vi "Measurement UI.vi"() -> ()   [LabVIEW 2025, in "TDMS Waveform Creator UI.lvlib"]
uses:
  TDMS Waveform Creator UI.lvlib
panel:
  out "Wfm List Item When Drag Start":i32
  out "Waveform Preview (Canvas)":waveform(dbl)(graph)
  in  "Waveform List":i32(listbox)
  in  "Duration":dbl=0.002 format="%#_6ps"
  in  "Sample Rate":dbl=10000000.0 caption="Sample Rate (Resampled)" format="%#_6pHz"
  in  "Add to Save":bool
  in  "Clear All":bool
  in  "Waveforms Summary JSON":string[](array[string])
  out "Waveform Preview (To Save)":waveform(dbl)[](graph)
  out "Channels Item When Drag Start":i32
  out "Max Sample Rate":dbl format="%#_6pHz"
  in  "Channel Names":string[](array[string])
  in  "Run Action":string(combo)="Create/Replace Wfm Group"
  in  "TDMS File Location":path
  in  "Wfm Group Name":string="Wfm1"
  in  "Channels":i32(listbox)
  # "Canvas"
  # "Waveform Group to Save"
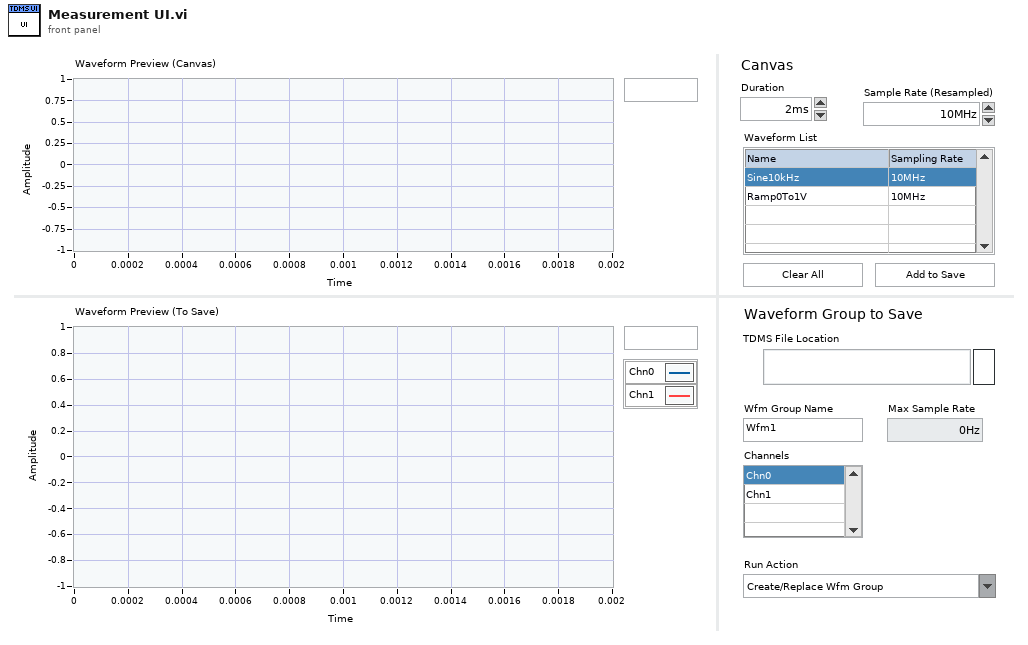
[diagram p1: front panel]
types:
  T1 = cluster{"Canvas Wfm Array":waveform(dbl)[], "To Save Wfm Arrays":waveform(dbl)[]}
  T2 = cluster{"Channels":refnum<vi>, "Channel Names":refnum<vi>, "Waveform Preview (To Save)":refnum<vi>, "Waveforms Summary JSON":refnum<vi>, "Max Sample Rate":refnum<vi>}
  T3 = cluster{"Waveform List":refnum<vi>, "Duration":refnum<vi>, "Sample Rate":refnum<vi>}
  T4 = enum16{"No Item", "1 Item", ">2 Item", "Invalid Selection"}
  T5 = typedef "LVPoint32TypeDef.ctl" = cluster{"Horizontal":i32, "Vertical":i32}
  T6 = typedef "LVRowAndColumnTypeDef.ctl" = cluster{"Row":i32, "Column":i32}
  T7 = cluster{"Canvas Wfm Array Out":waveform(dbl)[], "To Save Wfm Arrays":waveform(dbl)[]}
  T8 = cluster{"Channel Names":string[], "To Save Wfm Arrays Out":waveform(dbl)[], "Waveform Summary JSON":string[]}
  T9 = cluster{"Channel Names":string[], "To Save Wfm Arrays":waveform(dbl)[], "Waveform Summary JSON":string[]}
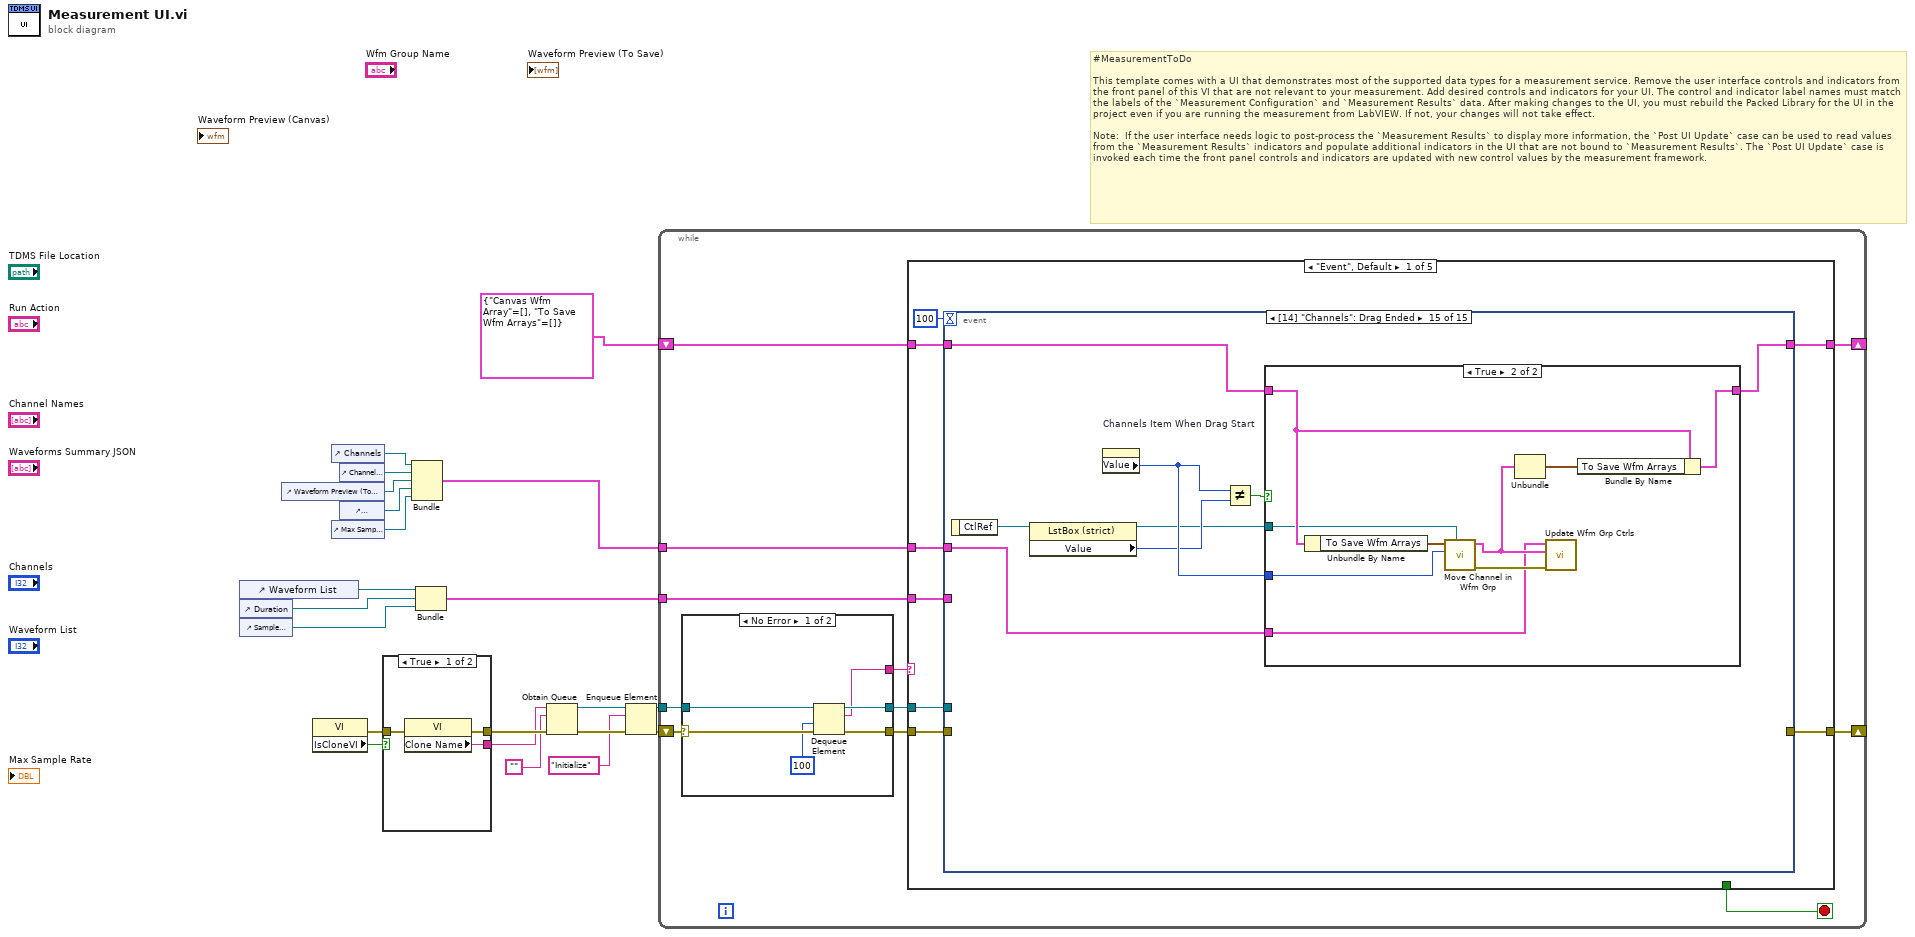
[diagram p0: block diagram]
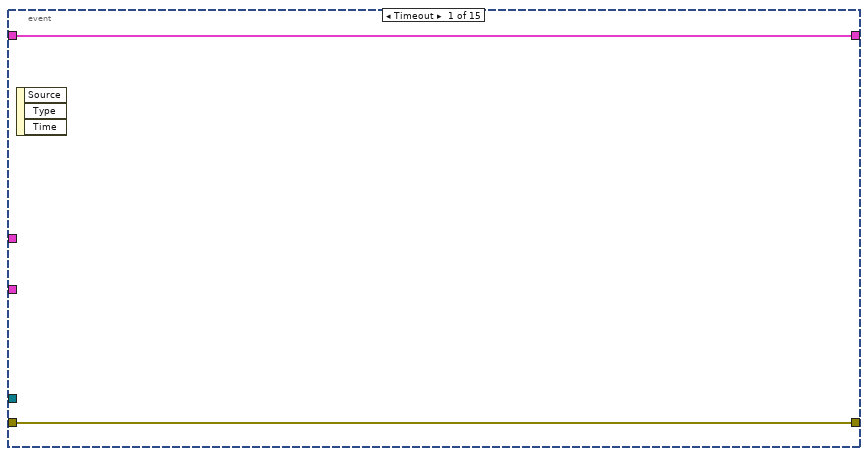
[diagram p2: hidden frame]
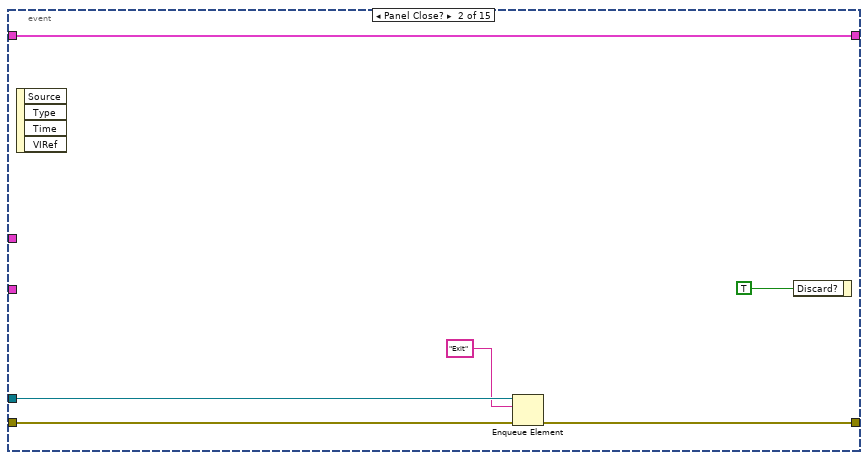
[diagram p3: hidden frame]
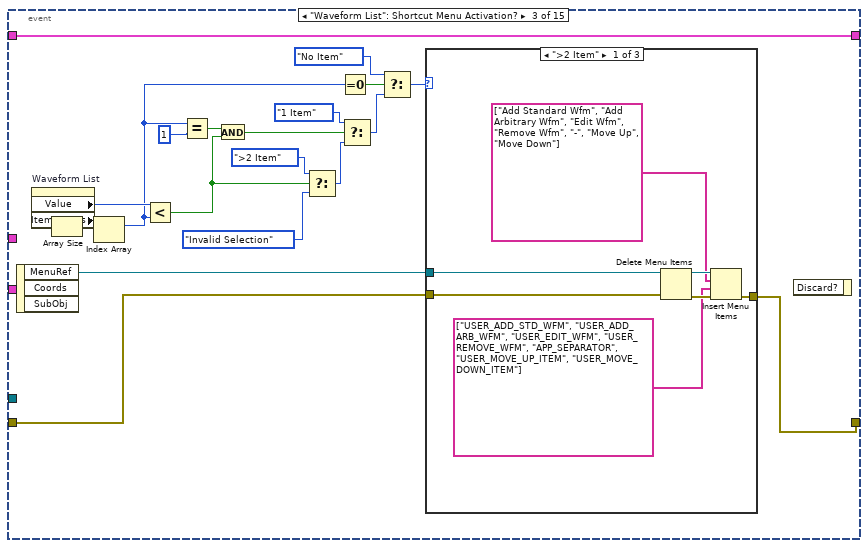
[diagram p4: hidden frame]
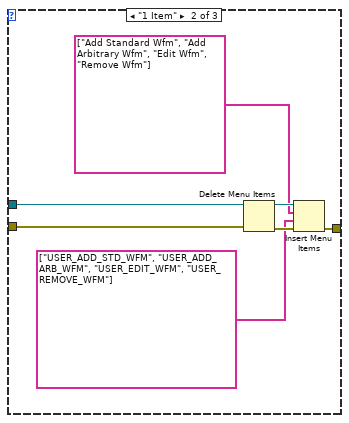
[diagram p5: hidden frame]
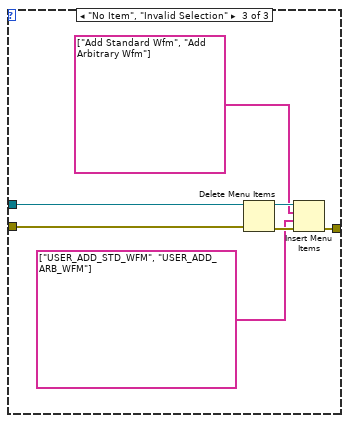
[diagram p6: hidden frame]
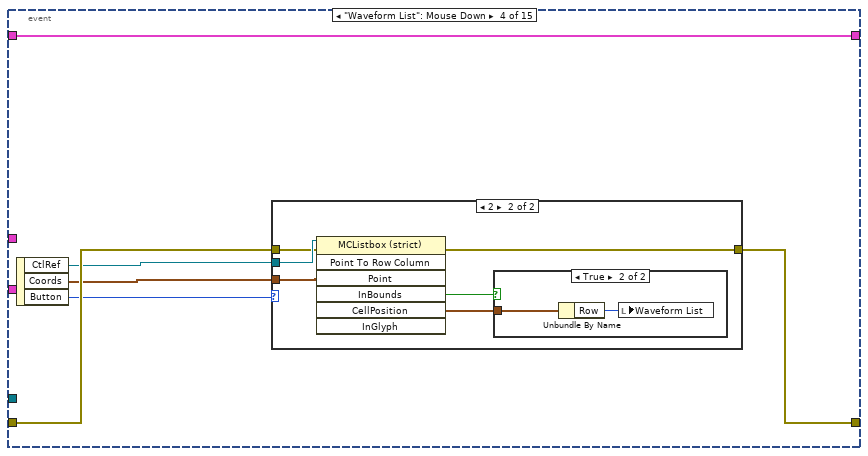
[diagram p7: hidden frame]
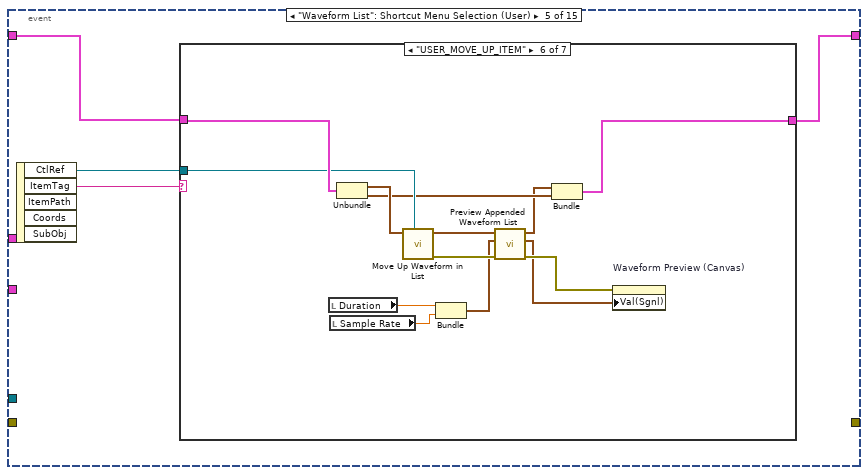
[diagram p10: hidden frame]
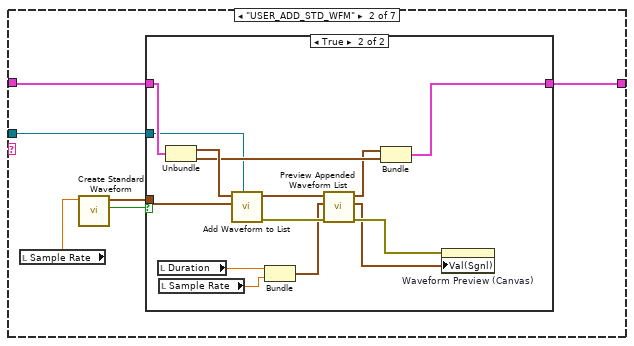
[diagram p12: hidden frame]
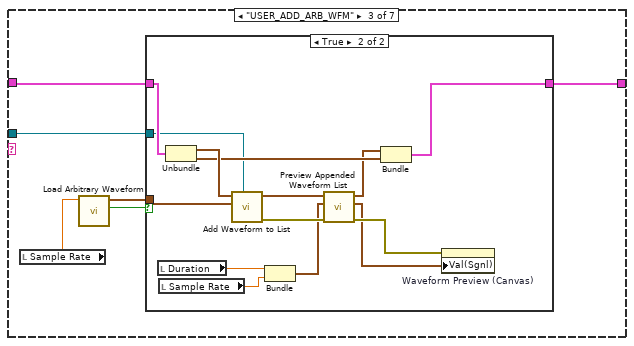
[diagram p14: hidden frame]
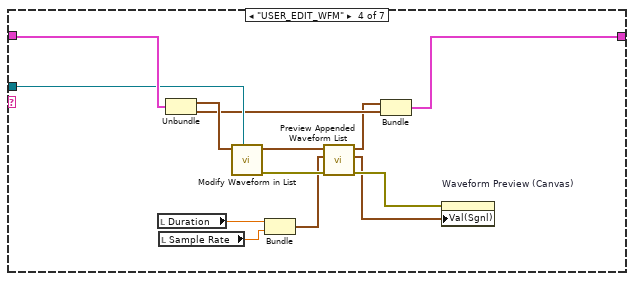
[diagram p16: hidden frame]
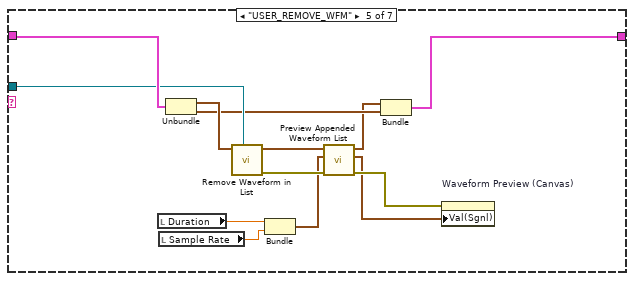
[diagram p17: hidden frame]
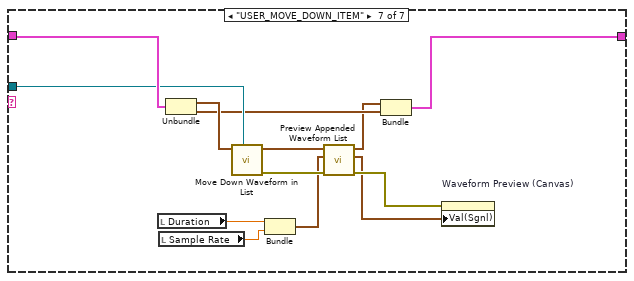
[diagram p18: hidden frame]
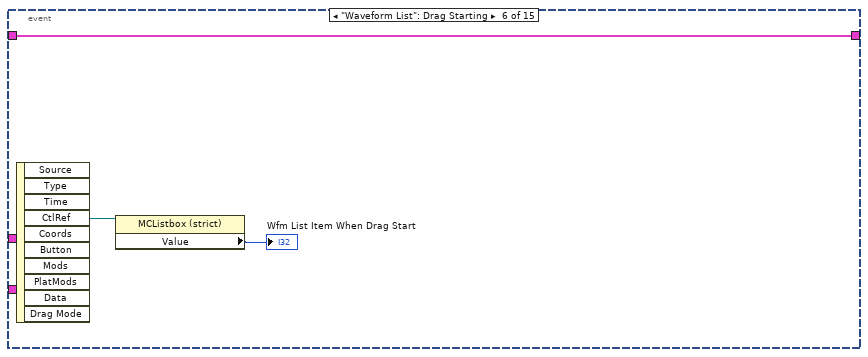
[diagram p19: hidden frame]
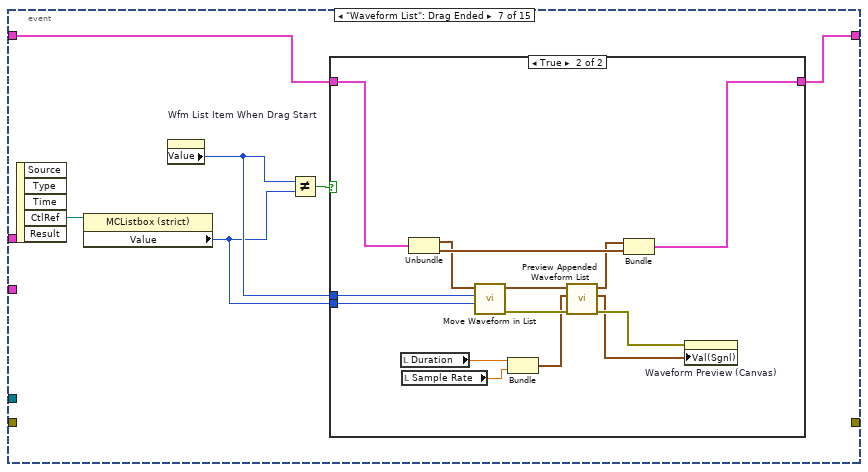
[diagram p20: hidden frame]
diagram:
  # "#MeasurementToDo  \n\nThis template comes with a UI that demonstrates most of the supported data types for a measurement service. Remove the user interface controls and indicators from the front panel of this VI that are not relevant to your measurement. Add desired controls and indicators for your UI. The control and indicator label names must match the labels of the `Measurement Configuration` and `Measurement Results` data. After making changes to the UI, you must rebuild the Packed Library for the UI in the project even if you are running the measurement from LabVIEW. If not, your changes will not take effect.\n\nNote:  If the user interface needs logic to post-process the `Measurement Results` to display more information, the `Post UI Update` case can be used to read values from the `Measurement Results` indicators and populate additional indicators in the UI that are not bound to `Measurement Results`. The `Post UI Update` case is invoked each time the front panel controls and indicators are updated with new control values by the measurement framework."
  n1 = control-ref of="Waveform List"() -> (w4:refnum<vi>)
  n2 = control-ref of="Duration"() -> (w5:refnum<vi>)
  n3 = control-ref of="Sample Rate"() -> (w6:refnum<vi>)
  n4 = control-ref of="Waveform Preview (To Save)"() -> (w8:refnum<vi>)
  n5 = property class="VI"() -> (error out=w12:errorcluster, "IsCloneVI"=w13:bool)  [unwired: 2 in, 1 out]
  n6 = control-ref of="Channels"() -> (w1:refnum<vi>)
  n7 = control-ref of="Max Sample Rate"() -> (w10:refnum<vi>)
  n8 = control-ref of="Channel Names"() -> (w7:refnum<vi>)
  n9 = control-ref of="Waveforms Summary JSON"() -> (w9:refnum<vi>)
  n10 = case shown="True" w13 {
    tunnel: [w24 w27] -> w21
    tunnel: [w23 w26] -> w20
    tunnel: w12 -> [w22 w25]
    frame True {
      n11 = property class="VI"(error in=w22) -> (error out=w24:errorcluster, "Clone Name"=w23:string)  [unwired: 1 in, 1 out]
    }
    frame False {
      n12 = property class="VI"(error in=w25) -> (error out=w27:errorcluster, "Name"=w26:string)  [unwired: 1 in, 1 out]
    }
  }
  n13 = Bundle("Channels"=w1, "Channel Names"=w7, "Waveform Preview (To Save)"=w8, "Waveforms Summary JSON"=w9, "Max Sample Rate"=w10) -> (w3:T2)  [unwired: 1 in]
  n14 = Bundle("Waveform List"=w4, "Duration"=w5, "Sample Rate"=w6) -> (w2:T3)  [unwired: 1 in]
  n15 = Obtain Queue(name (unnamed)=w20, element data type="", error in (no error)=w21) -> (queue out=w17:refnum<queue>, error out=w19:errorcluster)  [unwired: 2 in, 1 out]
  n16 = Enqueue Element(queue=w17, element="Initialize", error in (no error)=w19) -> (queue out=w16:refnum<queue>, error out=w18:errorcluster)  [unwired: 1 in, 1 out]
  n17 = while {
    shift-right: [w33] -> _
    shift-left: w18 -> [w38]
    tunnel: w16 -> [w36]
    shift-right: [w31] -> _
    shift-left: T1 {"Canvas Wfm Array"=[], "To Save Wfm Arrays"=[]} -> [w30]
    tunnel: w3 -> [w29]
    tunnel: w2 -> [w28]
    stop <- w32 stop-if-true
    n18 = case shown="No Error" w38 {
      selector: w38 -> [w459 w462]
      tunnel: [w458 w462] -> w37
      tunnel: w36 -> [w457 w461]
      tunnel: [w456 w461] -> w35
      tunnel: [w455 "Handle Error"] -> w34
      frame No Error {
        n19 = Dequeue Element(queue=w457, timeout in ms (-1)=100, error in (no error)=w459) -> (queue out=w456:refnum<queue>, element=w455:string, error out=w458:errorcluster)  [unwired: 1 out]
      }
      frame Error {
      }
    }
    n20 = case shown="\"Event\", Default" w34 {
      tunnel: w37 -> [w45 w433 w438 w451 w453]
      tunnel: w35 -> [w43 _ _ w449 _]
      tunnel: [w46 w429 w442 w446 w453] -> w33
      tunnel: [_ FALSE _ TRUE _] -> w32
      tunnel: [w42 w430 w440 w444 w452] -> w31
      tunnel: w30 -> [w41 w430 w443 w444 w452]
      tunnel: w29 -> [w40 _ w441 _ _]
      tunnel: w28 -> [w39 _ _ _ _]
      frame "Event", Default {
        n21 = event shown="[14] \"Channels\": Drag Ended" {
          selector: _ -> [_ _ _ _ _ _ _ _ _ _ _ _ _ _ _]
          dyn-events: _ -> [_ _ _ _ _ _ _ _ _ _ _ _ _ _ _]
          timeout: 100 -> [_ _ _ _ _ _ _ _ _ _ _ _ _ _ _]
          tunnel: [w48 w52 w73 w97 _ _ _ w236 w246 w259 w299 w324 w341 _ _] -> w46
          tunnel: w45 -> [w48 w53 w74 w101 _ _ _ w235 w245 w263 w300 w328 w339 _ _]
          tunnel: w43 -> [_ w51 _ _ _ _ _ _ _ _ _ _ _ _ _]
          tunnel: [w47 w49 w72 w96 w112 w212 w215 w239 w254 w264 w298 w323 w342 w410 w415] -> w42
          tunnel: w41 -> [w47 w49 w72 w96 w111 w212 w216 w239 w255 w262 w298 w323 w340 w410 w416]
          tunnel: w40 -> [_ _ _ _ _ _ _ _ _ w256 _ _ w338 _ w412]
          tunnel: w39 -> [_ _ _ _ _ _ _ _ _ _ _ _ w337 _ _]
          event Timeout {
            n22 = event-data() -> ()  [unwired: 1 in, 3 out]
          }
          event Panel Close? {
            n23 = event-data() -> ()  [unwired: 1 in, 4 out]
            n24 = Enqueue Element(queue=w51, element="Exit", error in (no error)=w53) -> (error out=w52:errorcluster)  [unwired: 1 in, 2 out]
            n25 = event-data("Discard?"=TRUE) -> ()  [unwired: 1 in, 1 out]
          }
          event "Waveform List": Shortcut Menu Activation? {
            n26 = event-data() -> ("MenuRef"=w68:refnum<k9>)  [unwired: 1 in, 2 out]
            n27 = property on="Waveform List" class="MCListbox (strict)"() -> ("Value"=w70:i32, "ItemNames"=w71:string[][])  [unwired: 2 in, 2 out]
            n28 = Array Size(array=w71) -> (size(s)=w69:i32[])
            n29 = Index Array(array=w69) -> (element=w64:i32)  [unwired: 1 in]
            n30 = Less?(x=w70, y=w64) -> (x < y?=w57:bool)
            n31 = Equal?(x=w64, y=1) -> (x = y?=w62:bool)
            n32 = And(x=w62, y=w57) -> (x .and. y?=w61:bool)
            n33 = Select(t=T4.">2 Item", s=w57, f=T4."Invalid Selection") -> (s? t:f=w59:T4)
            n34 = Equal To 0?(x=w64) -> (x = 0?=w67:bool)
            n35 = Select(t=T4."1 Item", s=w61, f=w59) -> (s? t:f=w56:T4)
            n36 = Select(t=T4."No Item", s=w67, f=w56) -> (s? t:f=w55:T4)
            n37 = case shown="\">2 Item\"" w55 {
              tunnel: w74 -> [w77 w84 w91]
              tunnel: [w76 w83 w90] -> w73
              tunnel: w68 -> [w75 w82 w89]
              frame ">2 Item" {
                n38 = Delete Menu Items(6:w77, 9:w75) -> (0:w81:errorcluster, 3:w80:refnum<k9>)  [unwired: 2 in]
                n39 = Insert Menu Items(6:w81, 7:string[] ["USER_ADD_STD_WFM", "USER_ADD_ARB_WFM", "USER_EDIT_WFM", "USER_REMOVE_WFM", "APP_SEPARATOR", "USER_MOVE_UP_ITEM", "USER_MOVE_DOWN_ITEM"], 8:string[] ["Add Standard Wfm", "Add Arbitrary Wfm", "Edit Wfm", "Remove Wfm", "-", "Move Up", "Move Down"], 9:w80) -> (0:w76:errorcluster)  [unwired: 2 in, 2 out]
              }
              frame "1 Item" {
                n40 = Delete Menu Items(6:w84, 9:w82) -> (0:w88:errorcluster, 3:w87:refnum<k9>)  [unwired: 2 in]
                n41 = Insert Menu Items(6:w88, 7:string[] ["USER_ADD_STD_WFM", "USER_ADD_ARB_WFM", "USER_EDIT_WFM", "USER_REMOVE_WFM"], 8:string[] ["Add Standard Wfm", "Add Arbitrary Wfm", "Edit Wfm", "Remove Wfm"], 9:w87) -> (0:w83:errorcluster)  [unwired: 2 in, 2 out]
              }
              frame "No Item", "Invalid Selection" {
                n42 = Delete Menu Items(6:w91, 9:w89) -> (0:w95:errorcluster, 3:w94:refnum<k9>)  [unwired: 2 in]
                n43 = Insert Menu Items(6:w95, 7:string[] ["USER_ADD_STD_WFM", "USER_ADD_ARB_WFM"], 8:string[] ["Add Standard Wfm", "Add Arbitrary Wfm"], 9:w94) -> (0:w90:errorcluster)  [unwired: 2 in, 2 out]
              }
            }
            n44 = event-data() -> ()  [unwired: 2 in, 1 out]
          }
          event "Waveform List": Mouse Down {
            n45 = event-data() -> ("CtlRef"=w100:refnum<vi>, "Coords"=w99:T5, "Button"=w98:u16)  [unwired: 1 in]
            n46 = case shown="2" w98 {
              tunnel: w99 -> [_ w108]
              tunnel: w100 -> [_ w107]
              tunnel: w101 -> [w102 w105]
              tunnel: [w102 w106] -> w97
              frame Default {
              }
              frame 2 {
                n47 = invoke class="MCListbox (strict)" method="Point To Row Column"(reference=w107, error in=w105, "Point"=w108) -> (error out=w106:errorcluster, "InBounds"=w103:bool, "CellPosition"=w104:T6)  [unwired: 4 in, 4 out]
                n48 = case shown="True" w103 {
                  tunnel: w104 -> [_ w110]
                  frame False {
                  }
                  frame True {
                    n49 = Unbundle By Name(w110) -> ("Row"=w109:i32)
                    n50 = local write "Waveform List"(w109) -> ()
                  }
                }
              }
            }
          }
          event "Waveform List": Shortcut Menu Selection (User) {
            n51 = event-data() -> ("CtlRef"=w113:refnum<vi>, "ItemTag"=w114:string)  [unwired: 1 in, 3 out]
            n52 = case shown="\"USER_MOVE_UP_ITEM\"" w114 {
              tunnel: w113 -> [_ w117 w138 w168 w181 w194 w207]
              tunnel: [w115 w121 w142 w170 w183 w196 w209] -> w112
              tunnel: w111 -> [w115 w118 w139 w169 w182 w195 w208]
              frame Default {
              }
              frame "USER_ADD_STD_WFM" {
                n53 = local read "Sample Rate"() -> (w116:dbl)
                n54 = call "Create Standard Waveform.vi"("Suggested Sample Rate (Hz)"=w116) -> ("Waveform Created?"=w120:bool, "Output Waveform"=w119:waveform(dbl))  [unwired: 9 in]
                n55 = case shown="True" w120 {
                  tunnel: [w122 w133] -> w121
                  tunnel: w119 -> [_ w136]
                  tunnel: w118 -> [w122 w135]
                  tunnel: w117 -> [_ w129]
                  frame False {
                  }
                  frame True {
                    n56 = local read "Duration"() -> (w131:dbl)
                    n57 = local read "Sample Rate"() -> (w130:dbl)
                    n58 = Unbundle(w135) -> ("Canvas Wfm Array"=w134:waveform(dbl)[], "To Save Wfm Arrays"=w132:waveform(dbl)[])
                    n59 = call "Add Waveform to List.vi"("Waveform List Ctl Ref"=w129, "Waveform to Add"=w136, "Canvas Wfm Array In"=w134) -> ("error out"=w128:errorcluster, "Canvas Wfm Array Out"=w126:waveform(dbl)[])  [unwired: 7 in]
                    n60 = Bundle("Duration"=w131, "Sample Rate"=w130) -> (w123:cluster{"Duration":dbl, "Sample Rate":dbl})  [unwired: 1 in]
                    n61 = call "Preview Appended Waveform List.vi"("error in (no error)"=w128, "Trim and Resample Settings"=w123, "Canvas Wfm Array In"=w126) -> ("error out"=w127:errorcluster, "Final Waveform"=w124:waveform(dbl), "Canvas Wfm Array Out"=w125:waveform(dbl)[])  [unwired: 6 in]
                    n62 = Bundle("Canvas Wfm Array Out"=w125, "To Save Wfm Arrays"=w132) -> (w133:T7)  [unwired: 1 in]
                    n63 = property on="Waveform Preview (Canvas)" class="WFGraph (strict)"(error in=w127, "Val(Sgnl)"=w124) -> ()  [unwired: 1 in, 2 out]
                  }
                }
              }
              frame "USER_ADD_ARB_WFM" {
                n64 = local read "Sample Rate"() -> (w137:dbl)
                n65 = call "Load Arbitrary Waveform.vi"("Suggested Sample Rate"=w137) -> ("Waveform Created?"=w141:bool, "Output Waveform"=w140:waveform(dbl))  [unwired: 9 in]
                n66 = case shown="True" w141 {
                  tunnel: [w143 w154] -> w142
                  tunnel: w140 -> [_ w157]
                  tunnel: w139 -> [w143 w156]
                  tunnel: w138 -> [_ w150]
                  frame False {
                  }
                  frame True {
                    n67 = local read "Duration"() -> (w152:dbl)
                    n68 = local read "Sample Rate"() -> (w151:dbl)
                    n69 = Unbundle(w156) -> ("Canvas Wfm Array"=w155:waveform(dbl)[], "To Save Wfm Arrays"=w153:waveform(dbl)[])
                    n70 = call "Add Waveform to List.vi"("Waveform List Ctl Ref"=w150, "Waveform to Add"=w157, "Canvas Wfm Array In"=w155) -> ("error out"=w149:errorcluster, "Canvas Wfm Array Out"=w147:waveform(dbl)[])  [unwired: 7 in]
                    n71 = Bundle("Duration"=w152, "Sample Rate"=w151) -> (w144:cluster{"Duration":dbl, "Sample Rate":dbl})  [unwired: 1 in]
                    n72 = call "Preview Appended Waveform List.vi"("error in (no error)"=w149, "Trim and Resample Settings"=w144, "Canvas Wfm Array In"=w147) -> ("error out"=w148:errorcluster, "Final Waveform"=w145:waveform(dbl), "Canvas Wfm Array Out"=w146:waveform(dbl)[])  [unwired: 6 in]
                    n73 = Bundle("Canvas Wfm Array Out"=w146, "To Save Wfm Arrays"=w153) -> (w154:T7)  [unwired: 1 in]
                    n74 = property on="Waveform Preview (Canvas)" class="WFGraph (strict)"(error in=w148, "Val(Sgnl)"=w145) -> ()  [unwired: 1 in, 2 out]
                  }
                }
              }
              frame "USER_EDIT_WFM" {
                n75 = local read "Duration"() -> (w165:dbl)
                n76 = local read "Sample Rate"() -> (w164:dbl)
                n77 = Unbundle(w169) -> ("Canvas Wfm Array"=w167:waveform(dbl)[], "To Save Wfm Arrays"=w166:waveform(dbl)[])
                n78 = call "Modify Waveform in List.vi"("Waveform List Ctl Ref"=w168, "Canvas Wfm Array In"=w167) -> ("error out"=w163:errorcluster, "Canvas Wfm Array Out"=w161:waveform(dbl)[])  [unwired: 8 in]
                n79 = Bundle("Duration"=w165, "Sample Rate"=w164) -> (w158:cluster{"Duration":dbl, "Sample Rate":dbl})  [unwired: 1 in]
                n80 = call "Preview Appended Waveform List.vi"("error in (no error)"=w163, "Trim and Resample Settings"=w158, "Canvas Wfm Array In"=w161) -> ("error out"=w162:errorcluster, "Final Waveform"=w159:waveform(dbl), "Canvas Wfm Array Out"=w160:waveform(dbl)[])  [unwired: 6 in]
                n81 = Bundle("Canvas Wfm Array Out"=w160, "To Save Wfm Arrays"=w166) -> (w170:T7)  [unwired: 1 in]
                n82 = property on="Waveform Preview (Canvas)" class="WFGraph (strict)"(error in=w162, "Val(Sgnl)"=w159) -> ()  [unwired: 1 in, 2 out]
              }
              frame "USER_REMOVE_WFM" {
                n83 = local read "Duration"() -> (w178:dbl)
                n84 = local read "Sample Rate"() -> (w177:dbl)
                n85 = Unbundle(w182) -> ("Canvas Wfm Array"=w180:waveform(dbl)[], "To Save Wfm Arrays"=w179:waveform(dbl)[])
                n86 = call "Remove Waveform in List.vi"("Waveform List Ctl Ref"=w181, "Canvas Wfm Array In"=w180) -> ("error out"=w176:errorcluster, "Canvas Wfm Array Out"=w174:waveform(dbl)[])  [unwired: 8 in]
                n87 = Bundle("Duration"=w178, "Sample Rate"=w177) -> (w171:cluster{"Duration":dbl, "Sample Rate":dbl})  [unwired: 1 in]
                n88 = call "Preview Appended Waveform List.vi"("error in (no error)"=w176, "Trim and Resample Settings"=w171, "Canvas Wfm Array In"=w174) -> ("error out"=w175:errorcluster, "Final Waveform"=w172:waveform(dbl), "Canvas Wfm Array Out"=w173:waveform(dbl)[])  [unwired: 6 in]
                n89 = Bundle("Canvas Wfm Array Out"=w173, "To Save Wfm Arrays"=w179) -> (w183:T7)  [unwired: 1 in]
                n90 = property on="Waveform Preview (Canvas)" class="WFGraph (strict)"(error in=w175, "Val(Sgnl)"=w172) -> ()  [unwired: 1 in, 2 out]
              }
              frame "USER_MOVE_UP_ITEM" {
                n91 = local read "Duration"() -> (w191:dbl)
                n92 = local read "Sample Rate"() -> (w190:dbl)
                n93 = Unbundle(w195) -> ("Canvas Wfm Array"=w193:waveform(dbl)[], "To Save Wfm Arrays"=w192:waveform(dbl)[])
                n94 = call "Move Up Waveform in List.vi"("Waveform List Ctl Ref"=w194, "Canvas Wfm Array In"=w193) -> ("error out"=w189:errorcluster, "Canvas Wfm Array Out"=w187:waveform(dbl)[])  [unwired: 8 in]
                n95 = Bundle("Duration"=w191, "Sample Rate"=w190) -> (w184:cluster{"Duration":dbl, "Sample Rate":dbl})  [unwired: 1 in]
                n96 = call "Preview Appended Waveform List.vi"("error in (no error)"=w189, "Trim and Resample Settings"=w184, "Canvas Wfm Array In"=w187) -> ("error out"=w188:errorcluster, "Final Waveform"=w185:waveform(dbl), "Canvas Wfm Array Out"=w186:waveform(dbl)[])  [unwired: 6 in]
                n97 = Bundle("Canvas Wfm Array Out"=w186, "To Save Wfm Arrays"=w192) -> (w196:T7)  [unwired: 1 in]
                n98 = property on="Waveform Preview (Canvas)" class="WFGraph (strict)"(error in=w188, "Val(Sgnl)"=w185) -> ()  [unwired: 1 in, 2 out]
              }
              frame "USER_MOVE_DOWN_ITEM" {
                n99 = local read "Duration"() -> (w204:dbl)
                n100 = local read "Sample Rate"() -> (w203:dbl)
                n101 = Unbundle(w208) -> ("Canvas Wfm Array"=w206:waveform(dbl)[], "To Save Wfm Arrays"=w205:waveform(dbl)[])
                n102 = call "Move Down Waveform in List.vi"("Waveform List Ctl Ref"=w207, "Canvas Wfm Array In"=w206) -> ("error out"=w202:errorcluster, "Canvas Wfm Array Out"=w200:waveform(dbl)[])  [unwired: 8 in]
                n103 = Bundle("Duration"=w204, "Sample Rate"=w203) -> (w197:cluster{"Duration":dbl, "Sample Rate":dbl})  [unwired: 1 in]
                n104 = call "Preview Appended Waveform List.vi"("error in (no error)"=w202, "Trim and Resample Settings"=w197, "Canvas Wfm Array In"=w200) -> ("error out"=w201:errorcluster, "Final Waveform"=w198:waveform(dbl), "Canvas Wfm Array Out"=w199:waveform(dbl)[])  [unwired: 6 in]
                n105 = Bundle("Canvas Wfm Array Out"=w199, "To Save Wfm Arrays"=w205) -> (w209:T7)  [unwired: 1 in]
                n106 = property on="Waveform Preview (Canvas)" class="WFGraph (strict)"(error in=w201, "Val(Sgnl)"=w198) -> ()  [unwired: 1 in, 2 out]
              }
            }
          }
          event "Waveform List": Drag Starting {
            n107 = event-data() -> ("CtlRef"=w211:refnum<vi>)  [unwired: 1 in, 9 out]
            n108 = property class="MCListbox (strict)"(reference=w211) -> ("Value"=→"Wfm List Item When Drag Start":i32)  [unwired: 1 in, 2 out]
          }
          event "Waveform List": Drag Ended {
            n109 = event-data() -> ("CtlRef"=w218:refnum<vi>)  [unwired: 1 in, 4 out]
            n110 = property class="MCListbox (strict)"(reference=w218) -> ("Value"=w213:i32)  [unwired: 1 in, 2 out]
            n111 = property on="Wfm List Item When Drag Start" class="DigNum (strict)"() -> ("Value"=w214:i32)  [unwired: 2 in, 2 out]
            n112 = Not Equal?(x=w214, y=w213) -> (x != y?=w217:bool)
            n113 = case shown="True" w217 {
              tunnel: w216 -> [w219 w224]
              tunnel: [w219 w223] -> w215
              tunnel: w214 -> [_ w221]
              tunnel: w213 -> [_ w220]
              frame False {
              }
              frame True {
                n114 = local read "Duration"() -> (w232:dbl)
                n115 = local read "Sample Rate"() -> (w231:dbl)
                n116 = Unbundle(w224) -> ("Canvas Wfm Array"=w222:waveform(dbl)[], "To Save Wfm Arrays"=w233:waveform(dbl)[])
                n117 = call "Move Waveform in List.vi"("After Move Index"=w220, "Before Move Index"=w221, "Canvas Wfm Array In"=w222) -> ("error out"=w230:errorcluster, "Canvas Wfm Array Out"=w228:waveform(dbl)[])  [unwired: 7 in]
                n118 = Bundle("Duration"=w232, "Sample Rate"=w231) -> (w225:cluster{"Duration":dbl, "Sample Rate":dbl})  [unwired: 1 in]
                n119 = call "Preview Appended Waveform List.vi"("error in (no error)"=w230, "Trim and Resample Settings"=w225, "Canvas Wfm Array In"=w228) -> ("error out"=w229:errorcluster, "Final Waveform"=w226:waveform(dbl), "Canvas Wfm Array Out"=w227:waveform(dbl)[])  [unwired: 6 in]
                n120 = Bundle("Canvas Wfm Array Out"=w227, "To Save Wfm Arrays"=w233) -> (w223:T7)  [unwired: 1 in]
                n121 = property on="Waveform Preview (Canvas)" class="WFGraph (strict)"(error in=w229, "Val(Sgnl)"=w226) -> ()  [unwired: 1 in, 2 out]
              }
            }
          }
          event "Sample Rate", "Duration": Value Change {
            n122 = event-data() -> ()  [unwired: 1 in, 6 out]
            n123 = Unbundle By Name(w239) -> ("Canvas Wfm Array"=w242:waveform(dbl)[])
            n124 = Bundle("Duration"="Duration", "Sample Rate"="Sample Rate") -> (w234:cluster{"Duration":dbl, "Sample Rate":dbl})  [unwired: 1 in]
            n125 = call "Preview Appended Waveform List.vi"("error in (no error)"=w235, "Trim and Resample Settings"=w234, "Canvas Wfm Array In"=w242) -> ("error out"=w241:errorcluster, "Final Waveform"=w240:waveform(dbl))  [unwired: 6 in, 1 out]
            n126 = property on="Waveform Preview (Canvas)" class="WFGraph (strict)"(error in=w241, "Val(Sgnl)"=w240) -> (error out=w236:errorcluster)  [unwired: 1 in, 1 out]
          }
          event "Clear All": Value Change {
            n127 = event-data() -> ()  [unwired: 1 in, 6 out]
            n128 = property on="Duration" class="DigNum (strict)"() -> ("Value"=w247:dbl)  [unwired: 2 in, 2 out]
            n129 = property on="Sample Rate" class="DigNum (strict)"() -> ("Value"=w248:dbl)  [unwired: 2 in, 2 out]
            n130 = property on="Waveform List" class="MCListbox (strict)"(error in=w245, "ItemNames"=string[][] [] ("Item Names")) -> (error out=w244:errorcluster)  [unwired: 1 in, 1 out]
            n131 = Bundle("Value"=w247, "Value"=w248) -> (w243:cluster{"Value":dbl, "Value":dbl})  [unwired: 1 in]
            n132 = call "Preview Appended Waveform List.vi"("error in (no error)"=w244, "Trim and Resample Settings"=w243, "Canvas Wfm Array In"=waveform(dbl)[] [] ("Canvas Wfm Array")) -> ("error out"=w252:errorcluster, "Final Waveform"=w251:waveform(dbl), "Canvas Wfm Array Out"=w250:waveform(dbl)[])  [unwired: 6 in]
            n133 = Bundle By Name(cluster=w255, "Canvas Wfm Array"=w250) -> (w254:T1)
            n134 = property on="Waveform Preview (Canvas)" class="WFGraph (strict)"(error in=w252, "Val(Sgnl)"=w251) -> (error out=w246:errorcluster)  [unwired: 1 in, 1 out]
          }
          event "Add to Save": Value Change {
            n135 = event-data() -> ()  [unwired: 1 in, 1 out]
            n136 = Unbundle By Name(w262) -> ("To Save Wfm Arrays"=w260:waveform(dbl)[], "Canvas Wfm Array"=w261:waveform(dbl)[])
            n137 = property on="Waveform List" class="MCListbox (strict)"() -> ("ItemNames"=w258:string[][])  [unwired: 2 in, 2 out]
            n138 = Empty Array?(array=w258) -> (empty?=w257:bool)
            n139 = case shown="False" w257 {
              tunnel: [w272 w281] -> w264
              tunnel: w263 -> [w278 w282]
              tunnel: w262 -> [w277 w281]
              tunnel: w261 -> [w275 _]
              tunnel: w260 -> [w276 _]
              tunnel: [w270 w282] -> w259
              tunnel: w256 -> [w265 _]
              frame False {
                n140 = property on="Duration" class="DigNum (strict)"() -> ("Value"=w279:dbl)  [unwired: 2 in, 2 out]
                n141 = property on="Sample Rate" class="DigNum (strict)"() -> ("Value"=w280:dbl)  [unwired: 2 in, 2 out]
                n142 = Bundle("Value"=w279, "Value"=w280) -> (w274:cluster{"Value":dbl, "Value":dbl})  [unwired: 1 in]
                n143 = control-ref of="Channels"() -> (w273:refnum<vi>)
                n144 = call "Add Canvas Wfm To Save.vi"("Canvas Trim and Resample Settings"=w274, "error in (no error)"=w278, "Canvas Wfm Array"=w275, "To Save Wfm Arrays In"=w276, "Channels Ctrl Ref"=w273) -> ("error out"=w271:errorcluster, "Waveform Summary JSON"=w267:string[], "To Save Wfm Arrays Out"=w269:waveform(dbl)[], "Channel Names"=w268:string[])  [unwired: 3 in]
                n145 = Bundle("Channel Names"=w268, "To Save Wfm Arrays Out"=w269, "Waveform Summary JSON"=w267) -> (w266:T8)  [unwired: 1 in]
                n146 = Bundle By Name(cluster=w277, "To Save Wfm Arrays"=w269) -> (w272:T1)
                n147 = call "Update Wfm Grp Ctrls.vi"("error in (no error)"=w271, "Wfm Grp Data"=w266, "Ctrl Refs"=w265) -> ("error out"=w270:errorcluster)  [unwired: 8 in]
              }
              frame True {
              }
            }
          }
          event "Channels": Shortcut Menu Activation? {
            n148 = event-data() -> ("MenuRef"=w301:refnum<k9>)  [unwired: 1 in]
            n149 = property on="Channels" class="LstBox (strict)"() -> ("Value"=w285:i32, "Item Names"=w297:string[])  [unwired: 2 in, 2 out]
            n150 = Array Size(array=w297) -> (size(s)=w284:i32)
            n151 = Less?(x=w285, y=w284) -> (x < y?=w287:bool)
            n152 = Equal?(x=w284, y=1) -> (x = y?=w292:bool)
            n153 = And(x=w292, y=w287) -> (x .and. y?=w291:bool)
            n154 = Select(t=T4.">2 Item", s=w287, f=T4."Invalid Selection") -> (s? t:f=w289:T4)
            n155 = Equal To 0?(x=w284) -> (x = 0?=w296:bool)
            n156 = Select(t=T4."1 Item", s=w291, f=w289) -> (s? t:f=w286:T4)
            n157 = Select(t=T4."No Item", s=w296, f=w286) -> (s? t:f=w283:T4)
            n158 = case shown="\">2 Item\"" w283 {
              tunnel: w301 -> [w304 w311 w318]
              tunnel: w300 -> [w303 w310 w317]
              tunnel: [w302 w309 w316] -> w299
              frame ">2 Item" {
                n159 = Delete Menu Items(6:w303, 9:w304) -> (0:w308:errorcluster, 3:w307:refnum<k9>)  [unwired: 2 in]
                n160 = Insert Menu Items(6:w308, 7:string[] ["USER_RENAME_CHN", "USER_EDIT_CHN", "USER_REMOVE_CHN", "APP_SEPARATOR", "USER_MOVE_UP_ITEM", "USER_MOVE_DOWN_ITEM"], 8:string[] ["Rename Channel", "Edit In Canvas", "Remove Channel", "-", "Move Up", "Move Down"], 9:w307) -> (0:w302:errorcluster)  [unwired: 2 in, 2 out]
              }
              frame "1 Item" {
                n161 = Delete Menu Items(6:w310, 9:w311) -> (0:w315:errorcluster, 3:w314:refnum<k9>)  [unwired: 2 in]
                n162 = Insert Menu Items(6:w315, 7:string[] ["USER_RENAME_CHN", "USER_EDIT_CHN", "USER_REMOVE_CHN"], 8:string[] ["Rename Channel", "Edit In Canvas", "Remove Channel"], 9:w314) -> (0:w309:errorcluster)  [unwired: 2 in, 2 out]
              }
              frame "No Item", "Invalid Selection" {
                n163 = Delete Menu Items(6:w317, 9:w318) -> (0:w322:errorcluster, 3:w321:refnum<k9>)  [unwired: 2 in]
                n164 = Insert Menu Items(6:w322, 7:string[] [], 8:string[] [], 9:w321) -> (0:w316:errorcluster)  [unwired: 2 in, 2 out]
              }
            }
            n165 = event-data() -> ()  [unwired: 2 in, 1 out]
          }
          event "Channels": Mouse Down {
            n166 = event-data() -> ("CtlRef"=w327:refnum<vi>, "Coords"=w326:T5, "Button"=w325:u16)  [unwired: 1 in, 2 out]
            n167 = case shown="2" w325 {
              tunnel: w326 -> [_ w335]
              tunnel: w327 -> [_ w334]
              tunnel: w328 -> [w329 w332]
              tunnel: [w329 w333] -> w324
              frame Default {
              }
              frame 2 {
                n168 = invoke class="LstBox (strict)" method="Point To Row"(reference=w334, error in=w332, "Point"=w335) -> (error out=w333:errorcluster, "InBounds"=w330:bool, "Row"=w331:i32)  [unwired: 4 in, 4 out]
                n169 = case shown="True" w330 {
                  tunnel: w331 -> [_ w336]
                  frame False {
                  }
                  frame True {
                    n170 = local write "Channels"(w336) -> ()
                  }
                }
              }
            }
          }
          event "Channels": Shortcut Menu Selection (User) {
            n171 = event-data() -> ("CtlRef"=w343:refnum<vi>, "ItemTag"=w344:string)  [unwired: 1 in]
            n172 = case shown="\"USER_MOVE_UP_ITEM\"" w344 {
              tunnel: w343 -> [_ w355 w374 w384 w394 w406]
              tunnel: [w346 w348 w370 w380 w390 w402] -> w342
              tunnel: [w345 w353 w372 w382 w392 w404] -> w341
              tunnel: w338 -> [_ w350 w366 w376 w386 w397]
              tunnel: w340 -> [w346 w349 w371 w381 w391 w403]
              tunnel: w339 -> [w345 w347 w367 w377 w387 w399]
              tunnel: w337 -> [_ _ _ _ _ w396]
              frame Default {
              }
              frame "USER_RENAME_CHN" {
                n173 = Unbundle By Name(w349) -> ("To Save Wfm Arrays"=w356:waveform(dbl)[])
                n174 = call "Rename Channel.vi"("Channels Ctrl Ref"=w355, "error in (no error)"=w347, "To Save Wfm Arrays"=w356) -> ("error out"=w354:errorcluster, "Udpated Wfm Grp Data"=w351:T9, "Channel Renamed?"=w352:bool)  [unwired: 6 in]
                n175 = case shown="True" w352 {
                  tunnel: w354 -> [w357 w365]
                  tunnel: [w357 w364] -> w353
                  tunnel: w351 -> [_ w362]
                  tunnel: w350 -> [_ w359]
                  tunnel: w349 -> [w358 w363]
                  tunnel: [w358 w361] -> w348
                  frame False {
                  }
                  frame True {
                    n176 = Unbundle(w362) -> ("To Save Wfm Arrays"=w360:waveform(dbl)[])  [unwired: 2 out]
                    n177 = call "Update Wfm Grp Ctrls.vi"("error in (no error)"=w365, "Wfm Grp Data"=w362, "Ctrl Refs"=w359) -> ("error out"=w364:errorcluster)  [unwired: 8 in]
                    n178 = Bundle By Name(cluster=w363, "To Save Wfm Arrays"=w360) -> (w361:T1)
                  }
                }
              }
              frame "USER_REMOVE_CHN" {
                n179 = Unbundle By Name(w371) -> ("To Save Wfm Arrays"=w375:waveform(dbl)[])
                n180 = call "Remove Channel.vi"("Channels Ctrl Ref"=w374, "error in (no error)"=w367, "To Save Wfm Arrays"=w375) -> ("error out"=w373:errorcluster, "Wfm Grp Data"=w369:T9)  [unwired: 7 in]
                n181 = Unbundle(w369) -> ("To Save Wfm Arrays"=w368:waveform(dbl)[])  [unwired: 2 out]
                n182 = call "Update Wfm Grp Ctrls.vi"("error in (no error)"=w373, "Wfm Grp Data"=w369, "Ctrl Refs"=w366) -> ("error out"=w372:errorcluster)  [unwired: 8 in]
                n183 = Bundle By Name(cluster=w371, "To Save Wfm Arrays"=w368) -> (w370:T1)
              }
              frame "USER_MOVE_UP_ITEM" {
                n184 = Unbundle By Name(w381) -> ("To Save Wfm Arrays"=w385:waveform(dbl)[])
                n185 = call "Move Up Channel in Wfm Grp.vi"("Channels Ctrl Ref"=w384, "error in (no error)"=w377, "To Save Wfm Arrays"=w385) -> ("error out"=w383:errorcluster, "Wfm Grp Data"=w379:T9)  [unwired: 7 in]
                n186 = Unbundle(w379) -> ("To Save Wfm Arrays"=w378:waveform(dbl)[])  [unwired: 2 out]
                n187 = call "Update Wfm Grp Ctrls.vi"("error in (no error)"=w383, "Wfm Grp Data"=w379, "Ctrl Refs"=w376) -> ("error out"=w382:errorcluster)  [unwired: 8 in]
                n188 = Bundle By Name(cluster=w381, "To Save Wfm Arrays"=w378) -> (w380:T1)
              }
              frame "USER_MOVE_DOWN_ITEM" {
                n189 = Unbundle By Name(w391) -> ("To Save Wfm Arrays"=w395:waveform(dbl)[])
                n190 = call "Move Down Channel in Wfm Grp.vi"("Channels Ctrl Ref"=w394, "error in (no error)"=w387, "To Save Wfm Arrays"=w395) -> ("error out"=w393:errorcluster, "Wfm Grp Data"=w389:T9)  [unwired: 7 in]
                n191 = Unbundle(w389) -> ("To Save Wfm Arrays"=w388:waveform(dbl)[])  [unwired: 2 out]
                n192 = call "Update Wfm Grp Ctrls.vi"("error in (no error)"=w393, "Wfm Grp Data"=w389, "Ctrl Refs"=w386) -> ("error out"=w392:errorcluster)  [unwired: 8 in]
                n193 = Bundle By Name(cluster=w391, "To Save Wfm Arrays"=w388) -> (w390:T1)
              }
              frame "USER_EDIT_CHN" {
                n194 = Unbundle By Name(w403) -> ("To Save Wfm Arrays"=w407:waveform(dbl)[])
                n195 = call "Move Chn to Wfm Canvas.vi"("Channels Ctrl Ref"=w406, "error in (no error)"=w399, "Canvas Ctrl Refs"=w396, "To Save Wfm Arrays"=w407) -> ("error out"=w405:errorcluster, "Canvas Wfm Arrays"=w398:waveform(dbl)[], "Wfm Grp Data"=w401:T9)  [unwired: 5 in]
                n196 = Unbundle(w401) -> ("To Save Wfm Arrays"=w400:waveform(dbl)[])  [unwired: 2 out]
                n197 = call "Update Wfm Grp Ctrls.vi"("error in (no error)"=w405, "Wfm Grp Data"=w401, "Ctrl Refs"=w397) -> ("error out"=w404:errorcluster)  [unwired: 8 in]
                n198 = Bundle By Name(cluster=w403, "To Save Wfm Arrays"=w400, "Canvas Wfm Array"=w398) -> (w402:T1)
              }
            }
          }
          event "Channels": Drag Starting {
            n199 = event-data() -> ("CtlRef"=w409:refnum<vi>)  [unwired: 1 in, 9 out]
            n200 = property class="LstBox (strict)"(reference=w409) -> ("Value"=→"Channels Item When Drag Start":i32)  [unwired: 1 in, 2 out]
          }
          event "Channels": Drag Ended {
            n201 = event-data() -> ("CtlRef"=w418:refnum<vi>)  [unwired: 1 in]
            n202 = property class="LstBox (strict)"(reference=w418) -> (reference out=w411:refnum<vi>, "Value"=w413:i32)  [unwired: 1 in, 1 out]
            n203 = property on="Channels Item When Drag Start" class="DigNum (strict)"() -> ("Value"=w414:i32)  [unwired: 2 in, 2 out]
            n204 = Not Equal?(x=w414, y=w413) -> (x != y?=w417:bool)
            n205 = case shown="True" w417 {
              tunnel: w416 -> [w419 w424]
              tunnel: [w419 w423] -> w415
              tunnel: w414 -> [_ w420]
              tunnel: w412 -> [_ w422]
              tunnel: w411 -> [_ w421]
              frame False {
              }
              frame True {
                n206 = Unbundle By Name(w424) -> ("To Save Wfm Arrays"=w428:waveform(dbl)[])
                n207 = call "Move Channel in Wfm Grp.vi"("Channels Ctrl Ref"=w421, "Before Move Index"=w420, "To Save Wfm Arrays"=w428) -> ("error out"=w427:errorcluster, "Wfm Grp Data"=w426:T9)  [unwired: 7 in]
                n208 = Unbundle(w426) -> ("To Save Wfm Arrays"=w425:waveform(dbl)[])  [unwired: 2 out]
                n209 = call "Update Wfm Grp Ctrls.vi"("error in (no error)"=w427, "Wfm Grp Data"=w426, "Ctrl Refs"=w422) -> ()  [unwired: 8 in, 1 out]
                n210 = Bundle By Name(cluster=w424, "To Save Wfm Arrays"=w425) -> (w423:T1)
              }
            }
          }
        }
      }
      frame "Initialize" {
        # "To invoke Preview Waveform redrawn"
        n211 = property on="Duration" class="DigNum (strict)"(error in=w433) -> (error out=w432:errorcluster, "Value"=w434:dbl)  [unwired: 1 in, 1 out]
        n212 = property on="Waveform List" class="MCListbox (strict)"("ItemNames"=string[][] [] ("Item Names")) -> ()  [unwired: 2 in, 2 out]
        n213 = property on="Channels" class="LstBox (strict)"("Item Names"=string[] []) -> ()  [unwired: 2 in, 2 out]
        n214 = property on="Duration" class="DigNum (strict)"(error in=w432, "Val(Sgnl)"=w434) -> (error out=w429:errorcluster)  [unwired: 1 in, 1 out]
        n215 = property on="Waveform Preview (Canvas)" class="WFGraph (strict)"("Val(Sgnl)"=waveform(dbl) {"t0"=timestamp(0 s since 1904-01-01), "dt"=1.0, "Y"=[]} ("Value (Signaling)")) -> ()  [unwired: 2 in, 2 out]
      }
      frame "Post UI Update" {
        # "This case will be triggered, after framework updates the User interface with result values."
        n216 = call "Initialize Wfm Grp Ctrls.vi"("error in (no error)"=w438, "Ctrl Refs"=w441) -> ("error out"=w442:errorcluster, "To Save Wfm Arrays"=w439:waveform(dbl)[])  [unwired: 8 in]
        n217 = Bundle By Name(cluster=w443, "To Save Wfm Arrays"=w439) -> (w440:T1)
      }
      frame "Exit" {
        # "This case is triggered to close the User Interface from framework"
        n218 = Flush Queue(queue=w449, error in (no error)=w451) -> (queue out=w448:refnum<queue>, error out=w447:errorcluster)  [unwired: 1 out]
        n219 = Release Queue(queue=w448, force destroy? (F)=TRUE, error in (no error)=w447) -> (error out=w446:errorcluster)  [unwired: 2 out]
      }
      frame "Handle Error" {
      }
    }
  }
